vi "CreateLiveChartData.vi"(8 "Live SMU":enum16{"A", "B"}(ring), 9 "Live DUT":u32=1 min=1 step=1, 10 "Live Measure Value":enum16{"Voltage", "Current", "Resistance"}(ring), 11 "SMU":dbl[][](array[numeric])) -> (1 "Live SMU Chart Y Scale Name":string, 2 "Live SMU Units":enum16{"V", "A", "Ohm"}(ring), 3 "Live SMU Chart":dbl)   [LabVIEW 2012]
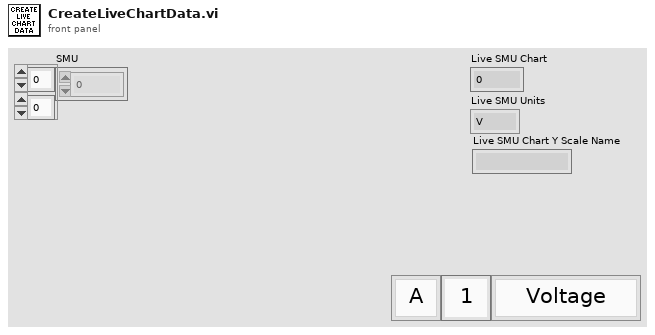
[diagram p1: front panel]
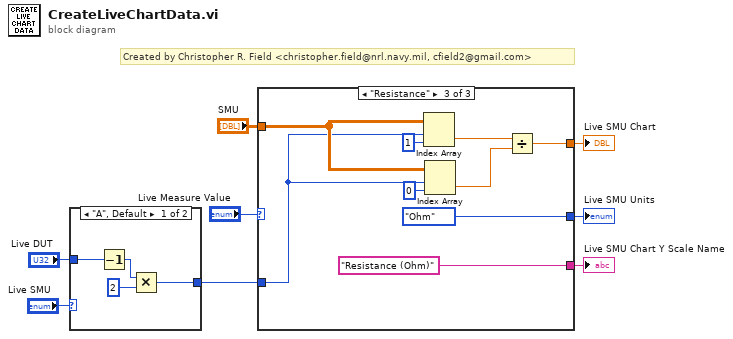
[diagram p0: block diagram]
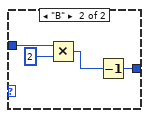
[diagram p2: hidden frame]
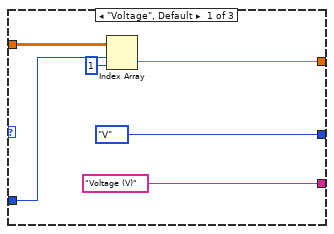
[diagram p3: hidden frame]
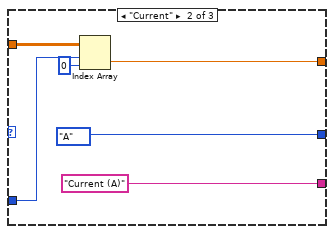
[diagram p4: hidden frame]
diagram:
  # "Created by Christopher R. Field <christopher.field@nrl.navy.mil, cfield2@gmail.com>"
  n1 = case shown="\"A\", Default" "Live SMU" {
    tunnel: [w9 w13] -> w5
    tunnel: "Live DUT" -> [w10 w16]
    frame "A", Default {
      n2 = Decrement(x=w10) -> (x-1=w11:u32)
      n3 = Multiply(x=w11, y=u32 2) -> (x*y=w9:u32)
    }
    frame "B" {
      n4 = Multiply(x=w16, y=u32 2) -> (x*y=w14:u32)
      n5 = Decrement(x=w14) -> (x-1=w13:u32)
    }
  }
  n6 = case shown="\"Resistance\"" "Live Measure Value" {
    tunnel: "SMU" -> [w22 w28 w33]
    tunnel: [w19 w27 w31] -> w3
    tunnel: w5 -> [w21 w26 w32]
    tunnel: [enum16{"V", "A", "Ohm"}."V" ("Chart Units") enum16{"V", "A", "Ohm"}."A" ("Chart Units") enum16{"V", "A", "Ohm"}."Ohm" ("Chart Units")] -> w2
    tunnel: ["Voltage (V)" ("Y Scale.Name Label.Text") "Current (A)" ("Y Scale.Name Label.Text") "Resistance (Ohm)" ("Y Scale.Name Label.Text")] -> w1
    frame "Voltage", Default {
      n7 = Index Array(array=w22, index (row)=w21, index (col)=1 ("disabled index (col)")) -> (element=w19:dbl)
    }
    frame "Current" {
      n8 = Index Array(array=w28, index (row)=w26, index (col)=0 ("disabled index (col)")) -> (element=w27:dbl)
    }
    frame "Resistance" {
      n9 = Index Array(array=w33, index (row)=w32, index (col)=1 ("disabled index (col)")) -> (element=w35:dbl)
      n10 = Index Array(array=w33, index (row)=w32, index (col)=0 ("disabled index (col)")) -> (element=w34:dbl)
      n11 = Divide(x=w35, y=w34) -> (x/y=w31:dbl)
    }
  }
  "Live SMU Chart" <- w3
  "Live SMU Units" <- w2
  "Live SMU Chart Y Scale Name" <- w1
